vi "NetComm_getControlWord.vi"(8 "error in (no error)":errorcluster) -> (0 "error out":errorcluster, 2 "Control Word":T1)   [LabVIEW 2017]
uses:
  <vilib>/Rock Robotics/SystemInterfaces/NetworkCommunication/NetComm_ControlWord.ctl
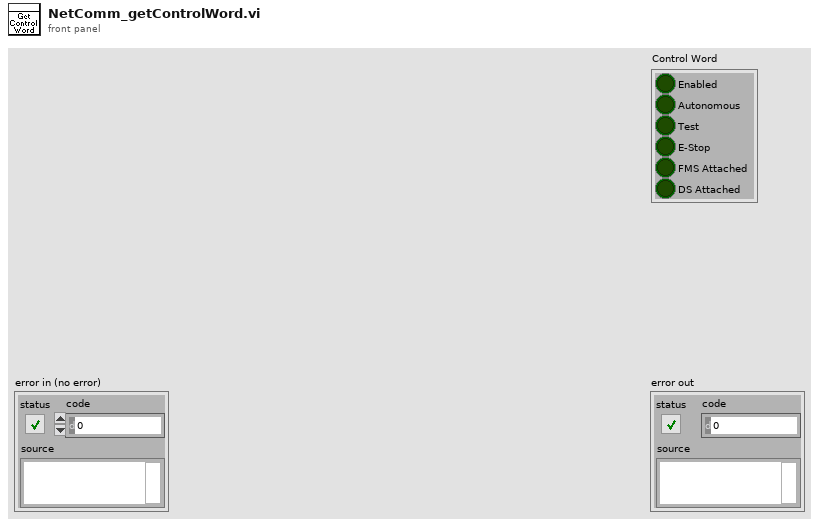
[diagram p1: front panel]
types:
  T1 = typedef "NetComm_ControlWord.ctl" = cluster{"Enabled":bool, "Autonomous":bool, "Test":bool, "E-Stop":bool, "FMS Attached":bool, "DS Attached":bool}
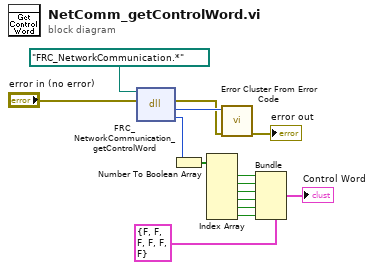
[diagram p0: block diagram]
diagram:
  n1 = dll-call lib="?" fn="FRC_NetworkCommunication_getControlWord"(path in=path "FRC_NetworkCommunication.*", error in="error in (no error)") -> (error out=w12:errorcluster, "return type"=w14:i32, "controlWord"=w9:u32)  [unwired: 2 in, 1 out]
  n2 = Number To Boolean Array(number=w9) -> (Boolean array=w8:bool[])
  n3 = Index Array(array=w8) -> (element #1=w7:bool, element #2=w6:bool, element #3=w5:bool, element #4=w3:bool, element #5=w4:bool, element #6=w1:bool)  [unwired: 6 in]
  n4 = call <vilib>:"Error Cluster From Error Code.vi"("error in (no error)"=w12, "error code (0)"=w14) -> ("error out"=→"error out":errorcluster)  [unwired: 7 in]
  n5 = Bundle(cluster=T1 {"Enabled"=FALSE, "Autonomous"=FALSE, "Test"=FALSE, "E-Stop"=FALSE, "FMS Attached"=FALSE, "DS Attached"=FALSE}, "Enabled"=w7, "Autonomous"=w6, "Test"=w5, "E-Stop"=w3, "FMS Attached"=w4, "DS Attached"=w1) -> (→"Control Word":T1)
